vi "GetPaneReference.vi"(8 "error in":errorcluster, 11 "Pane in":refnum<class "Pane.lvclass">) -> (0 "error out":errorcluster, 1 "pane reference":refnum<vi>, 3 "Pane out":refnum<class "Pane.lvclass">)   [LabVIEW 2014, in "Raspberry Pi Compatible Compiler for LabVIEW.lvlib" / "Pane.lvclass"]
uses:
  Pane.lvclass
  Generic/Generic.lvclass
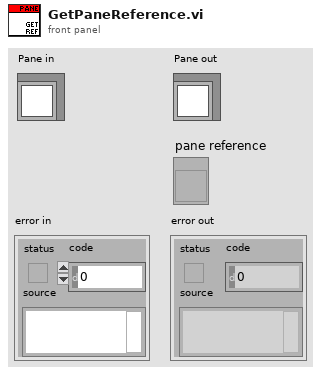
[diagram p1: front panel]
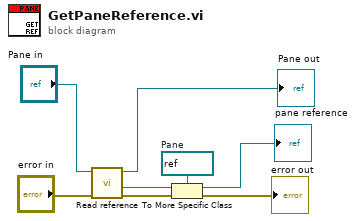
[diagram p0: block diagram]
diagram:
  w8 = refnum<vi> refnum  # Pane
  n1 = call "Read reference.vi"("error in"="error in", "GObject in"="Pane in") -> ("error out"=w7:errorcluster, "reference"=w6:refnum<vi>, "GObject out"=→"Pane out":refnum<class "Pane.lvclass">)  [unwired: 5 in]
  n2 = To More Specific Class(target class=w8, reference=w6, error in=w7) -> (specific class reference=→"pane reference":refnum<vi>, error out=→"error out":errorcluster)
